vi "Set Temperature.vi"(6 "Channel":i32, 8 "error in (no error)":errorcluster, 9 "Rate (K/min)":dbl, 10 "Temperature (K)":dbl, 11 "Instrument.Cryostat in":refnum<class "Instrument.Cryostat.lvclass">) -> (0 "error out":errorcluster, 3 "Instrument.Cryostat out":refnum<class "Instrument.Cryostat.lvclass">)   [LabVIEW 2019, in "Instrument.Cryostat.lvclass"]
uses:
  Instrument.Cryostat.lvclass
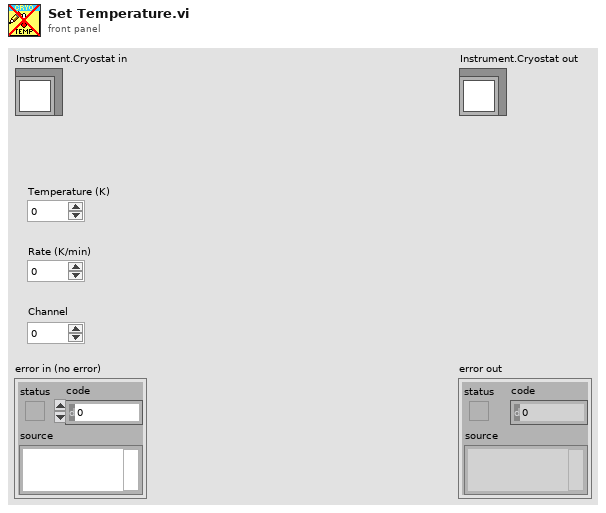
[diagram p1: front panel]
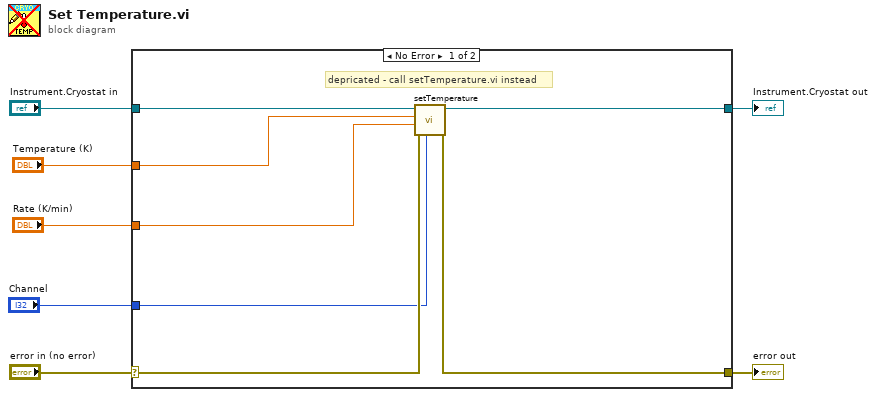
[diagram p0: block diagram]
diagram:
  n1 = case shown="No Error" "error in (no error)" {
    selector: "error in (no error)" -> [w14 w16]
    tunnel: [w11 w16] -> w6
    tunnel: [w13 w15] -> w4
    tunnel: "Instrument.Cryostat in" -> [w12 w15]
    tunnel: "Channel" -> [w10 _]
    tunnel: "Rate (K/min)" -> [w9 _]
    tunnel: "Temperature (K)" -> [w8 _]
    frame No Error {
      # "depricated - call setTemperature.vi instead"
      n2 = call-dynamic "setTemperature.vi"("Channel"=w10, "error in (no error)"=w14, "Rate (K/min)"=w9, "Temperature (K)"=w8, "Instrument.Cryostat in"=w12) -> ("error out"=w11:errorcluster, "Instrument.Cryostat out"=w13:refnum<class "Instrument.Cryostat.lvclass">)  [unwired: 5 in]
    }
    frame Error {
    }
  }
  "error out" <- w6
  "Instrument.Cryostat out" <- w4
